vi "AI_StreamingAI_MultipleChannels test v1.vi"() -> ()   [LabVIEW 2013]
uses:
  <vilib>/Platform/TimedLoop/XDataNode/timing_clust.ctl
  <vilib>/Platform/TimedLoop/XDataNode/nitl_modes.ctl
  <vilib>/Platform/TimedLoop/XDataNode/wakeup.ctl
  <userlib>/DAQNavi Polymorphic VI/create/DAQNavi Create Channel(AI-Voltage).vi
  <userlib>/DAQNavi Polymorphic VI/configure/timing/DAQNavi Timing(Convert Clock).vi
  <userlib>/DAQNavi Polymorphic VI/configure/DAQNavi Get Property/AI/DAQNaviGet_AI_ConvertClock_Rate.vi
  <userlib>/DAQNavi Polymorphic VI/read/DAQNavi Read (Analog 1D Wfm NChan NSamp).vi
  <vilib>/platform/TimedLoop/XDataNode/XDataNode.xnode
  <vilib>/Platform/TimedLoop/XDataNode/XDNodeRunTimeDep.lvlib
panel:
  out "Test":timestamp
  out "Start":timestamp
  out "loops":bool
  out "error out":errorcluster
  out "Waveform Graph":waveform(dbl)[](graph)
  out "value range":string="+/- 5 V" caption="property value"
  out "physical channels":string="DemoDevice,BID#0/ai0:1" caption="property value"
  in  "number of samples per channel to read":u32=1000
  in  "samples per channel":i32=1024
  out "actual convert rate":dbl
  in  "convert clock rate":dbl=1000.0
  out "overrun count":i32
  in  "stop":bool
  # "Please modify physical channels and value range in Channel Parameters\nthrough DAQNavi Property Assistant VI  in block diagram."
  # "Channel Parameters"
  # "Timing Parameters"
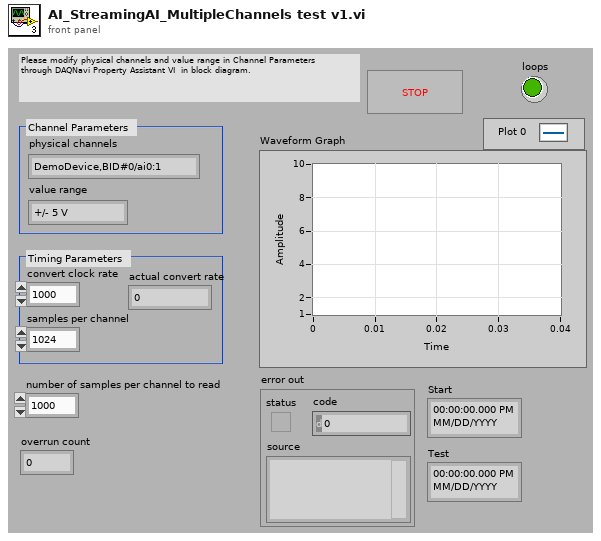
[diagram p1: front panel]
types:
  T1 = typedef "XDNodeRunTimeDep.lvlib/timing_clust.ctl" = cluster{"Expected End [f-1]":u64, "Actual End [f-1]":u64, "Finished Late? [f-1]":bool, "Expected End [i-1]":u64, "Actual End [i-1]":u64, "Finished Late? [i-1]":bool, "Expected Start [i]":u64, "Actual Start [i]":u64, "Expected Start [f]":u64, "Actual Start [f]":u64, "Source Name":string, "Structure Name":string, "Period":i64, "Deadline":i64, "Offset":i64, "Start":i64, "Priority":i32, "Timeout":i32, "Mode":T2, "Wakeup Reason":T3, "Error":errorcluster, "Source Type":string, "Secondary Source Type":string, "Global End Time":u64, "Global Start Time":u64, "Frame Duration":u64, "Iteration Duration":u64, "Assigned CPU":i32, "I/O Scan Engine Mode":u32}
  T2 = typedef "XDNodeRunTimeDep.lvlib/nitl_modes.ctl" = enum32{"No Change", "Process missed periods, maintain original phase", "Discard missed periods, maintain original phase", "Process missed periods, ignore original phase", "Discard missed periods, ignore original phase"}
  T3 = typedef "XDNodeRunTimeDep.lvlib/wakeup.ctl" = enum32{"Normal", "Aborted", "Asynchronous wakeup", "Timing source error", "Timed loop error", "Timeout"}
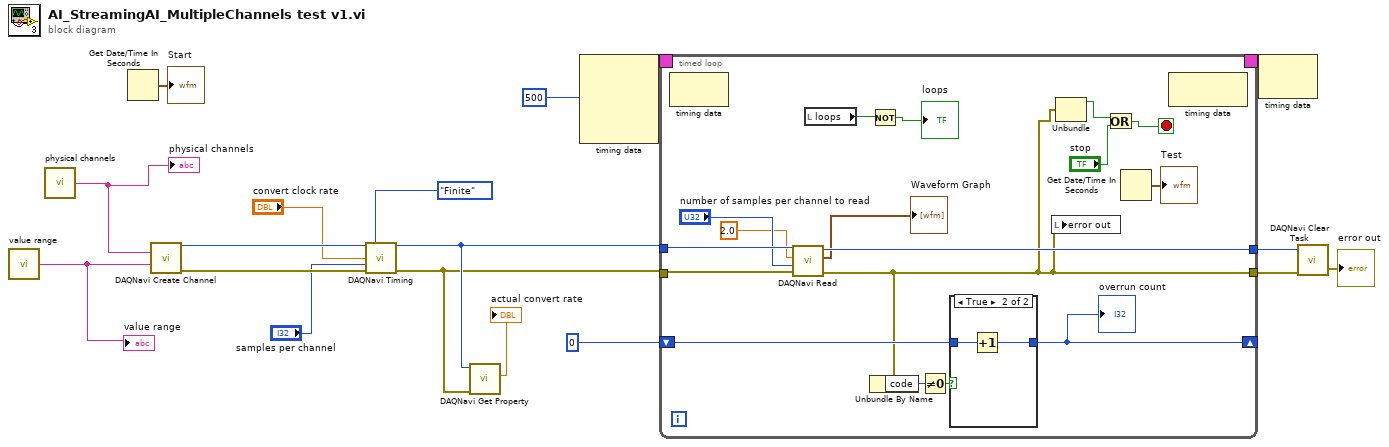
[diagram p0: block diagram]
diagram:
  n1 = call "value range"() -> ("property value"=w8:string)  [unwired: 1 out]
  "value range" <- w8
  n2 = call "physical channels"() -> ("property value"=w9:string)  [unwired: 1 out]
  "physical channels" <- w9
  n3 = Get Date/Time In Seconds() -> (seconds since 1Jan1904=→"Start":timestamp)
  n4 = call-poly <userlib>:"DAQNavi Create Channel.vi"("physical channels"=w9, "value range"=w8) -> ("task out"=w18:i32, "error out"=w17:errorcluster)  [unwired: 3 in, 9 out]
  n5 = call-poly <userlib>:"DAQNavi Timing.vi"("task in"=w18, "sample mode"=enum16{"Finite", "Continuous"}."Finite", "rate"="convert clock rate", "samples per channel"="samples per channel", "error in (no error)"=w17) -> ("task out"=w13:i32, "error out"=w12:errorcluster)  [unwired: 1 in, 8 out]
  n6 = call-poly <userlib>:"DAQNavi Get Property.vi"("error in (no error)"=w12, "task in"=w13) -> ("rate"=→"actual convert rate":dbl)  [unwired: 9 out]
  n7 = node-c288(500) -> (w4:T1)  [unwired: 3 in]
  n8 = timed-loop {
    tunnel: w13 -> [w34]
    tunnel: w12 -> [w35]
    shift-right: [w30] -> _
    shift-left: 0 -> [w31]
    tunnel: [w28] -> w7
    tunnel: [w24] -> w6
    timing: w4 -> [_]
    timing-out: [_] -> w3
    stop <- w21 stop-if-true
    n9 = node-c288() -> ()  [unwired: 1 in, 1 out]
    n10 = call-poly <userlib>:"DAQNavi Read.vi"("error in (no error)"=w35, "number of samples per channel to read"="number of samples per channel to read", "timeout"=2.0, "task in"=w34) -> ("error out"=w24:errorcluster, "data"=→"Waveform Graph":waveform(dbl)[], "task out"=w28:i32)  [unwired: 5 out]
    n11 = local read "loops"() -> (w26:bool)
    n12 = Not(x=w26) -> (.not. x?=→"loops":bool)
    n13 = Unbundle By Name(w24) -> ("code"=w33:i32)
    n14 = Not Equal To 0?(x=w33) -> (x != 0?=w32:bool)
    n15 = case shown="True" w32 {
      tunnel: w31 -> [w38 w40]
      tunnel: [w38 w39] -> w30
      frame False {
      }
      frame True {
        n16 = Increment(x=w40) -> (x+1=w39:i32)
      }
    }
    "overrun count" <- w30
    n17 = local write "error out"(w24) -> ()
    n18 = Unbundle(w24) -> ("status"=w23:bool)  [unwired: 2 out]
    n19 = Or(x=w23, y="stop") -> (x .or. y?=w21:bool)
    n20 = Get Date/Time In Seconds() -> (seconds since 1Jan1904=→"Test":timestamp)
    n21 = node-c288() -> ()  [unwired: 1 in, 1 out]
  }
  n22 = node-c288(w3) -> ()  [unwired: 1 out]
  n23 = call <userlib>:"DAQNavi Clear Task.vi"("error in (no error)"=w6, "task in"=w7) -> ("error out"=→"error out":errorcluster)  [unwired: 1 out]
